vi "BBB_BundleAuxData.vi"(10 "Data in":T2) -> (1 "Aux data to display":T1={"LED T"=0.0, "Sink T"=0.0, "TEC Current"=0.0, "TEC Voltage"=0.0, "Is LED T stable?"=FALSE, "Is TEC enabled?"=FALSE, "TEC Status"=enum."Error", "Cavity Flow"=0.0, "Cavity Flow Setpoint"=0.0, "Overflow"=0.0, "Overflow Setpoint"=0.0, "LED Current"=0.0, "Cavity Pressure"=0.0, "Cavity T"=0.0, "Box T"=0.0, "LED on/off"=FALSE, "ZA/He valve"=FALSE, "NO2 add valve"=FALSE}, 2 "Aux data to Plot":T3)   [LabVIEW 2025]
uses:
  TypeDef_AuxDataToPlot.ctl
  TypeDef_DataIn.ctl
  TypeDef_AuxDataToDisplay.ctl
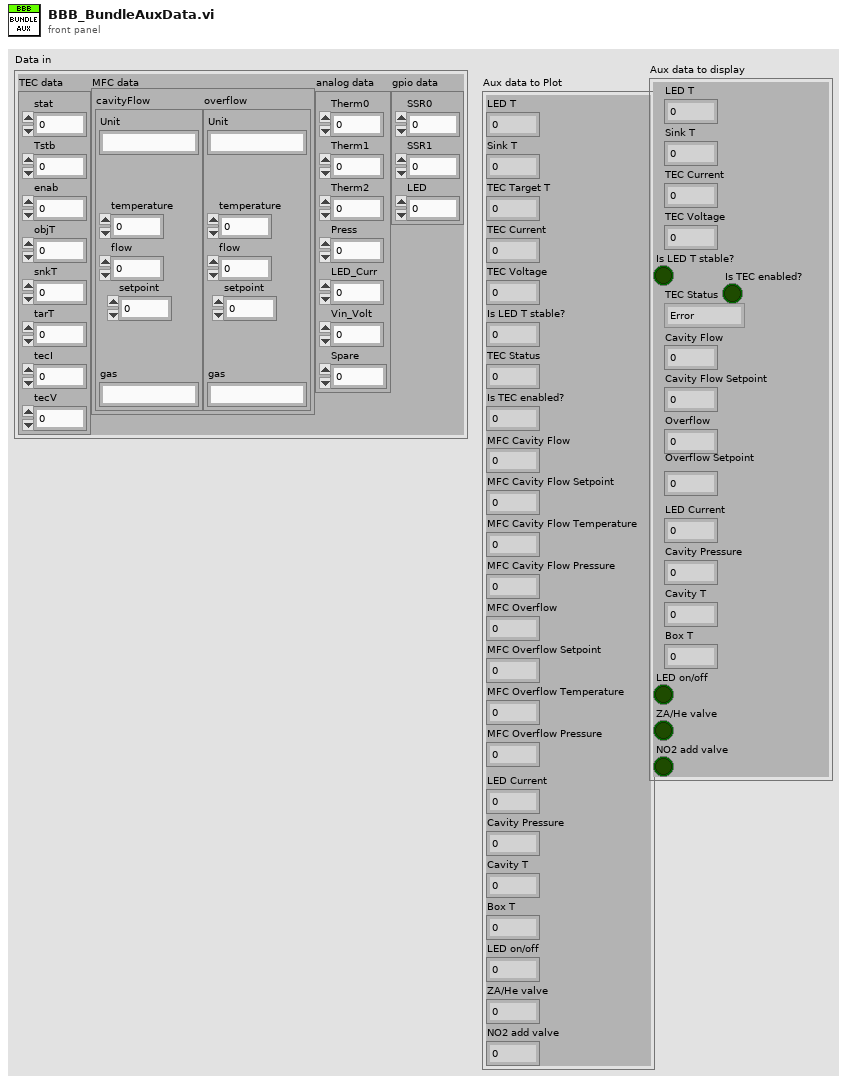
[diagram p1: front panel]
types:
  T1 = typedef "TypeDef_AuxDataToDisplay.ctl" = cluster{"LED T":dbl, "Sink T":dbl, "TEC Current":dbl, "TEC Voltage":dbl, "Is LED T stable?":bool, "Is TEC enabled?":bool, "TEC Status":enum16{"Initializing", "Idle", "Running", "Error", "Bootloader", "Device restarting"}, "Cavity Flow":dbl, "Cavity Flow Setpoint":dbl, "Overflow":dbl, "Overflow Setpoint":dbl, "LED Current":dbl, "Cavity Pressure":dbl, "Cavity T":dbl, "Box T":dbl, "LED on/off":bool, "ZA/He valve":bool, "NO2 add valve":bool}
  T2 = typedef "TypeDef_DataIn.ctl" = cluster{"TEC data":cluster{"stat":i32, "Tstb":i32, "enab":i32, "objT":dbl, "snkT":dbl, "tarT":dbl, "tecI":dbl, "tecV":dbl}, "MFC data":cluster{"cavityFlow":cluster{"Unit":string, "temperature":dbl, "flow":dbl, "setpoint":dbl, "gas":string}, "overflow":cluster{"Unit":string, "temperature":dbl, "flow":dbl, "setpoint":dbl, "gas":string}}, "analog data":cluster{"Therm0":dbl, "Therm1":dbl, "Therm2":dbl, "Press":dbl, "LED_Curr":dbl, "Vin_Volt":dbl, "Spare":dbl}, "gpio data":cluster{"SSR0":i32, "SSR1":i32, "LED":i32}}
  T3 = typedef "TypeDef_AuxDataToPlot.ctl" = cluster{"LED T":dbl, "Sink T":dbl, "TEC Target T":dbl, "TEC Current":dbl, "TEC Voltage":dbl, "Is LED T stable?":dbl, "TEC Status":dbl, "Is TEC enabled?":dbl, "MFC Cavity Flow":dbl, "MFC Cavity Flow Setpoint":dbl, "MFC Cavity Flow Temperature":dbl, "MFC Cavity Flow Pressure":dbl, "MFC Overflow":dbl, "MFC Overflow Setpoint":dbl, "MFC Overflow Temperature":dbl, "MFC Overflow Pressure ":dbl, "LED Current":dbl, "Cavity Pressure":dbl, "Cavity T":dbl, "Box T":dbl, "LED on/off":dbl, "ZA/He valve":dbl, "NO2 add valve":dbl}
  T4 = cluster{"stat":i32, "Tstb":i32, "enab":i32, "objT":dbl, "snkT":dbl, "tarT":dbl, "tecI":dbl, "tecV":dbl}
  T5 = cluster{"cavityFlow":cluster{"Unit":string, "temperature":dbl, "flow":dbl, "setpoint":dbl, "gas":string}, "overflow":cluster{"Unit":string, "temperature":dbl, "flow":dbl, "setpoint":dbl, "gas":string}}
  T6 = cluster{"Therm0":dbl, "Therm1":dbl, "Therm2":dbl, "Press":dbl, "LED_Curr":dbl, "Vin_Volt":dbl, "Spare":dbl}
  T7 = cluster{"Unit":string, "temperature":dbl, "flow":dbl, "setpoint":dbl, "gas":string}
  T8 = enum16{"Initializing", "Idle", "Running", "Error", "Bootloader", "Device restarting"}
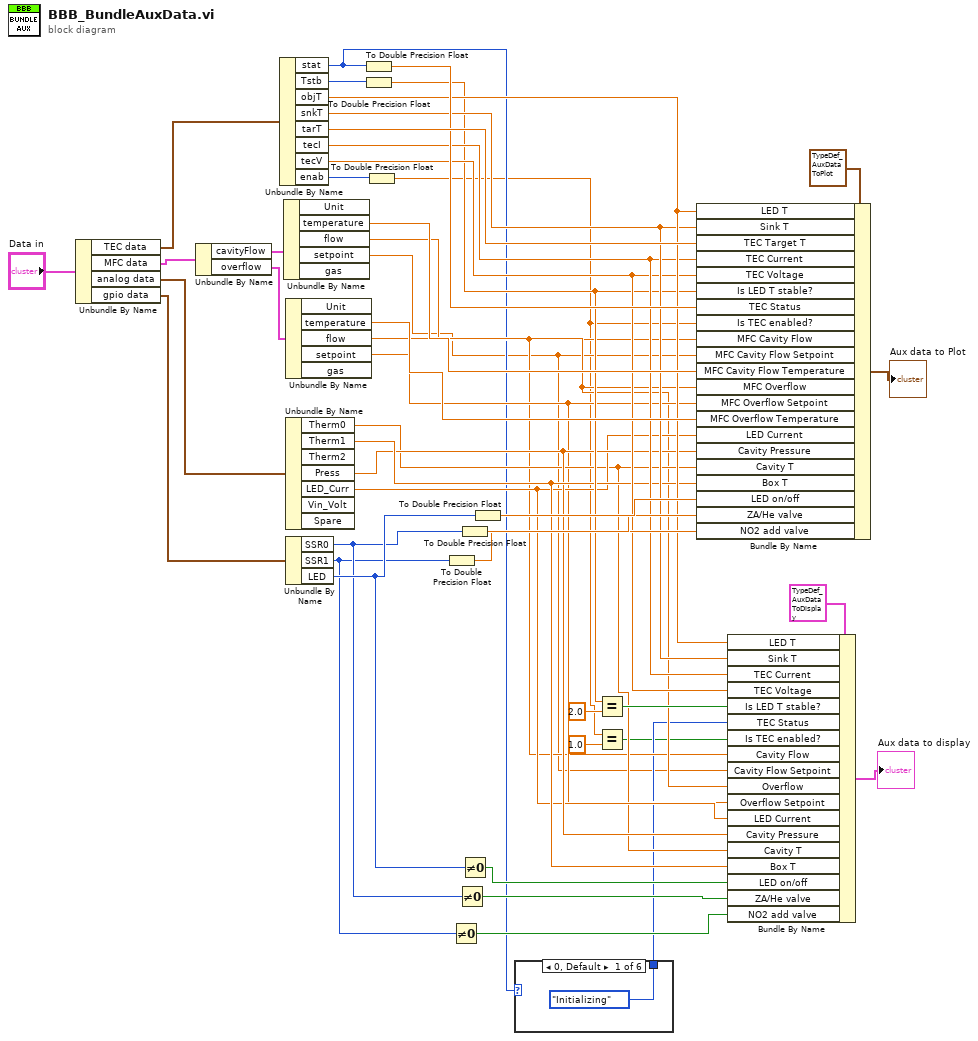
[diagram p0: block diagram]
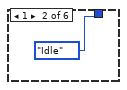
[diagram p2: hidden frame]
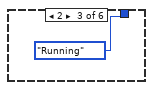
[diagram p3: hidden frame]
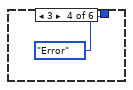
[diagram p4: hidden frame]
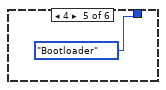
[diagram p5: hidden frame]
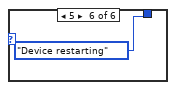
[diagram p6: hidden frame]
diagram:
  n1 = Unbundle By Name("Data in") -> ("TEC data"=w33:T4, "MFC data"=w32:T5, "analog data"=w31:T6, "gpio data"=w30:cluster{"SSR0":i32, "SSR1":i32, "LED":i32})
  n2 = Unbundle By Name(w32) -> ("cavityFlow"=w36:T7, "overflow"=w35:T7)
  n3 = Unbundle By Name(w33) -> ("stat"=w7:i32, "Tstb"=w45:i32, "objT"=w28:dbl, "snkT"=w27:dbl, "tarT"=w46:dbl, "tecI"=w26:dbl, "tecV"=w25:dbl, "enab"=w3:i32)
  n4 = Unbundle By Name(w36) -> ("temperature"=w40:dbl, "flow"=w9:dbl, "setpoint"=w5:dbl)  [unwired: 2 out]
  n5 = Unbundle By Name(w35) -> ("temperature"=w39:dbl, "flow"=w10:dbl, "setpoint"=w11:dbl)  [unwired: 2 out]
  n6 = Unbundle By Name(w31) -> ("Therm0"=w12:dbl, "Therm1"=w15:dbl, "Press"=w14:dbl, "LED_Curr"=w13:dbl)  [unwired: 3 out]
  n7 = Unbundle By Name(w30) -> ("SSR0"=w19:i32, "SSR1"=w17:i32, "LED"=w21:i32)
  n8 = To Double Precision Float(number=w7) -> (double precision float=w44:dbl)
  n9 = To Double Precision Float(number=w45) -> (double precision float=w23:dbl)
  n10 = To Double Precision Float(number=w3) -> (double precision float=w1:dbl)
  n11 = To Double Precision Float(number=w17) -> (double precision float=w41:dbl)
  n12 = Not Equal To 0?(x=w17) -> (x != 0?=w16:bool)
  n13 = Not Equal To 0?(x=w19) -> (x != 0?=w18:bool)
  n14 = To Double Precision Float(number=w19) -> (double precision float=w42:dbl)
  n15 = Not Equal To 0?(x=w21) -> (x != 0?=w20:bool)
  n16 = To Double Precision Float(number=w21) -> (double precision float=w43:dbl)
  n17 = case shown="0, Default" w7 {
    tunnel: [T8."Initializing" ("TEC Status") T8."Idle" ("TEC Status") T8."Running" ("TEC Status") T8."Error" ("TEC Status") T8."Bootloader" ("TEC Status") T8."Device restarting" ("TEC Status")] -> w6
    frame 0, Default {
    }
    frame 1 {
    }
    frame 2 {
    }
    frame 3 {
    }
    frame 4 {
    }
    frame 5 {
    }
  }
  n18 = Equal?(x=w23, y=2.0) -> (x = y?=w22:bool)
  n19 = Equal?(x=w1, y=1.0) -> (x = y?=w2:bool)
  n20 = Bundle By Name(cluster=T3 {"LED T"=0.0, "Sink T"=0.0, "TEC Target T"=0.0, "TEC Current"=0.0, "TEC Voltage"=0.0, "Is LED T stable?"=0.0, "TEC Status"=0.0, "Is TEC enabled?"=0.0, "MFC Cavity Flow"=0.0, "MFC Cavity Flow Setpoint"=0.0, "MFC Cavity Flow Temperature"=0.0, "MFC Cavity Flow Pressure"=0.0, "MFC Overflow"=0.0, "MFC Overflow Setpoint"=0.0, "MFC Overflow Temperature"=0.0, "MFC Overflow Pressure "=0.0, "LED Current"=0.0, "Cavity Pressure"=0.0, "Cavity T"=0.0, "Box T"=0.0, "LED on/off"=0.0, "ZA/He valve"=0.0, "NO2 add valve"=0.0} ("Aux data"), "LED T"=w28, "Sink T"=w27, "TEC Target T"=w46, "TEC Current"=w26, "TEC Voltage"=w25, "Is LED T stable?"=w23, "TEC Status"=w44, "Is TEC enabled?"=w1, "MFC Cavity Flow"=w9, "MFC Cavity Flow Setpoint"=w5, "MFC Cavity Flow Temperature"=w40, "MFC Overflow"=w10, "MFC Overflow Setpoint"=w11, "MFC Overflow Temperature"=w39, "LED Current"=w13, "Cavity Pressure"=w14, "Cavity T"=w12, "Box T"=w15, "LED on/off"=w43, "ZA/He valve"=w42, "NO2 add valve"=w41) -> (→"Aux data to Plot":T3)
  n21 = Bundle By Name(cluster=T1 {"LED T"=0.0, "Sink T"=0.0, "TEC Current"=0.0, "TEC Voltage"=0.0, "Is LED T stable?"=FALSE, "Is TEC enabled?"=FALSE, "TEC Status"=enum."Error", "Cavity Flow"=0.0, "Cavity Flow Setpoint"=0.0, "Overflow"=0.0, "Overflow Setpoint"=0.0, "LED Current"=0.0, "Cavity Pressure"=0.0, "Cavity T"=0.0, "Box T"=0.0, "LED on/off"=FALSE, "ZA/He valve"=FALSE, "NO2 add valve"=FALSE} ("Aux data"), "LED T"=w28, "Sink T"=w27, "TEC Current"=w26, "TEC Voltage"=w25, "Is LED T stable?"=w22, "TEC Status"=w6, "Is TEC enabled?"=w2, "Cavity Flow"=w9, "Cavity Flow Setpoint"=w5, "Overflow"=w10, "Overflow Setpoint"=w11, "LED Current"=w13, "Cavity Pressure"=w14, "Cavity T"=w12, "Box T"=w15, "LED on/off"=w20, "ZA/He valve"=w18, "NO2 add valve"=w16) -> (→"Aux data to display":T1)
